vi "Confirm-deposition.vi"(8 "error in (no error)":errorcluster, 10 "Succes? in":bool, 11 "Data Value Reference in":T1) -> (0 "error out":errorcluster, 2 "Succes?":bool, 3 "Data Value Reference out":T1)   [LabVIEW 2013, in "SLMControl.lvlib" / "SC-Main.lvclass"]
uses:
  SC-Main.lvclass
  Object-reference.ctl
  SC-Main.lvclass/SC-Main.ctl
  Read Deposition dialog.vi
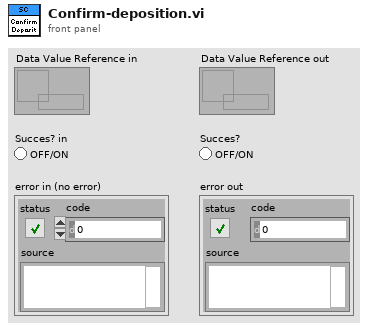
[diagram p1: front panel]
types:
  T1 = typedef "SLMControl.lvlib/SC-Main.lvclass/Object-reference.ctl" = refnum<data-value>
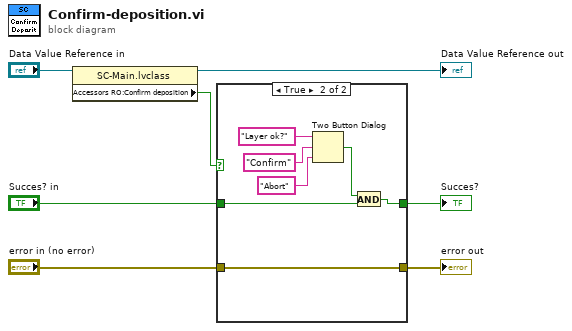
[diagram p0: block diagram]
diagram:
  n1 = property class="SC-Main.lvclass"(reference="Data Value Reference in") -> (reference out=→"Data Value Reference out":T1, "Accessors RO:Confirm deposition"=w7:bool)  [unwired: 1 in, 1 out]
  n2 = case shown="True" w7 {
    tunnel: "Succes? in" -> [w9 w16]
    tunnel: [w9 w15] -> w3
    tunnel: "error in (no error)" -> [w8 w12]
    tunnel: [w8 w12] -> w5
    frame False {
    }
    frame True {
      n3 = Two Button Dialog(message="Layer ok?", 1:"Abort" ("F button name (\"Cancel\")"), 2:"Confirm" ("T button name (\"OK\")")) -> (T button?=w13:bool)
      n4 = And(x=w13, y=w16) -> (x .and. y?=w15:bool)
    }
  }
  "error out" <- w5
  "Succes?" <- w3
